vi "funk.vi"() -> ()   [LabVIEW 2021]
panel:
  out "Y":dbl
  in  "X":dbl min=0.0 max=100.0 step=1.0
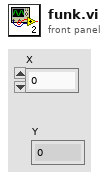
[diagram p1: front panel]
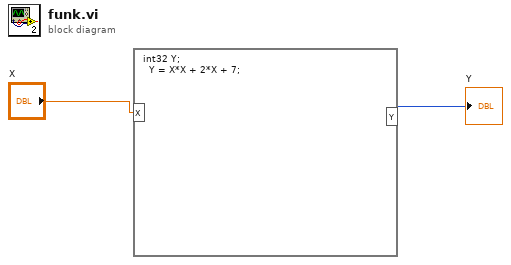
[diagram p0: block diagram]
diagram:
  n1 = formula code="int32 Y;\n\t\tY = X*X + 2*X + 7;"("X"="X") -> ("Y"=→"Y":i32)
